vi "LaserPIDPositioning.vi"(0 "Servo Device In":i32, 1 "Vertical Edge":T1 {"Point2 (Real-World)"."Y" format="%.2f"; "Point2 (Real-World)"."X" format="%.2f"; "Point1 (Real-World)"."Y" format="%.2f"; "Point1 (Real-World)"."X" format="%.2f"; "Point2 (Pixels)"."Y" format="%.2f"; "Point2 (Pixels)"."X" format="%.2f"; "Point1 (Pixels)"."Y" format="%.2f"; "Point1 (Pixels)"."X" format="%.2f"}, 2 "Horizontal Edge":T1 {"Point2 (Real-World)"."Y" format="%.2f"; "Point2 (Real-World)"."X" format="%.2f"; "Point1 (Real-World)"."Y" format="%.2f"; "Point1 (Real-World)"."X" format="%.2f"; "Point2 (Pixels)"."Y" format="%.2f"; "Point2 (Pixels)"."X" format="%.2f"; "Point1 (Pixels)"."Y" format="%.2f"; "Point1 (Pixels)"."X" format="%.2f"}, 4 "servo error in":errorcluster, 5 "error in":errorcluster, 8 "Destination Point":cluster{"DestinationX":dbl, "DestinationY":dbl}, 9 "Servo Angles In":cluster{"Angle X":dbl, "Angle Y":dbl}) -> (11 "Servo Angles Out":cluster{"Angle X":dbl, "Angle Y":dbl}, 14 "Servo Device Out":i32, 18 "servo error out":errorcluster, 19 "error out":errorcluster)   [LabVIEW 2014]
uses:
  <vilib>/addons/control/pid/pid.llb/PID (DBL).vi
  <vilib>/vision/NI_Vision_Development_Module.lvlib
  <vilib>/addons/control/pid/NI_PID_pid.lvlib
panel:
  out "x+y 2":dbl
  out "x+y":dbl
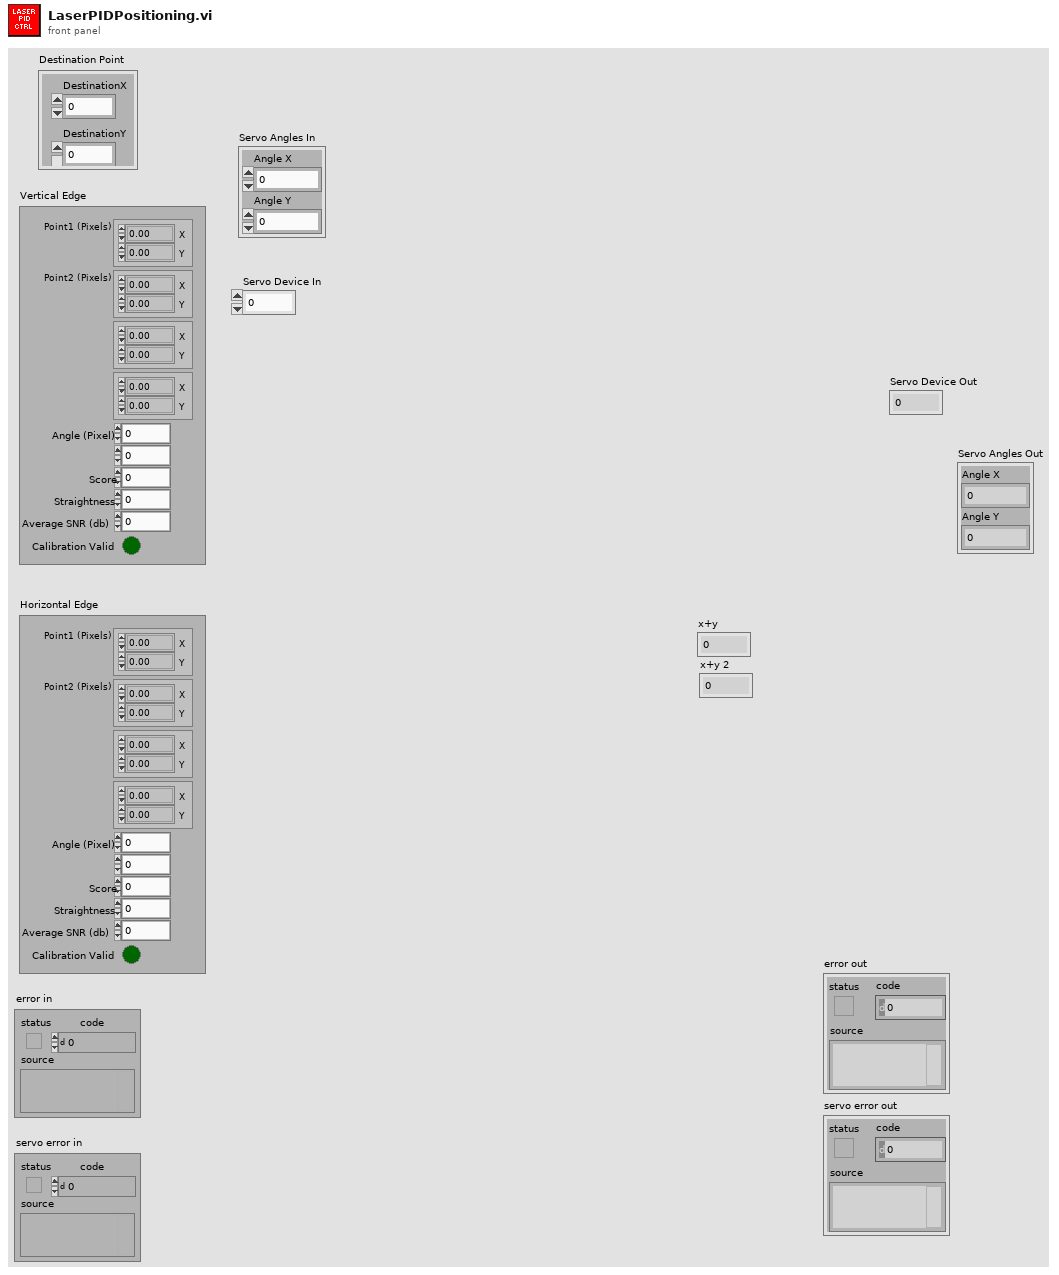
[diagram p1: front panel]
types:
  T1 = cluster{"Point1 (Pixels)":cluster{"X":sgl, "Y":sgl}, "Point2 (Pixels)":cluster{"X":sgl, "Y":sgl}, "Point1 (Real-World)":cluster{"X":sgl, "Y":sgl}, "Point2 (Real-World)":cluster{"X":sgl, "Y":sgl}, "Angle (Pixel)":dbl, "Angle (Real-World)":dbl, "Score":dbl, "Straightness":dbl, "Average SNR (db)":dbl, "Calibration Valid":bool}
  T2 = cluster{"proportional gain (Kc)":dbl, "integral time (Ti, min)":dbl, "derivative time (Td, min)":dbl}
  T3 = cluster{cluster{"X":sgl, "Y":sgl}, cluster{"X":sgl, "Y":sgl}}
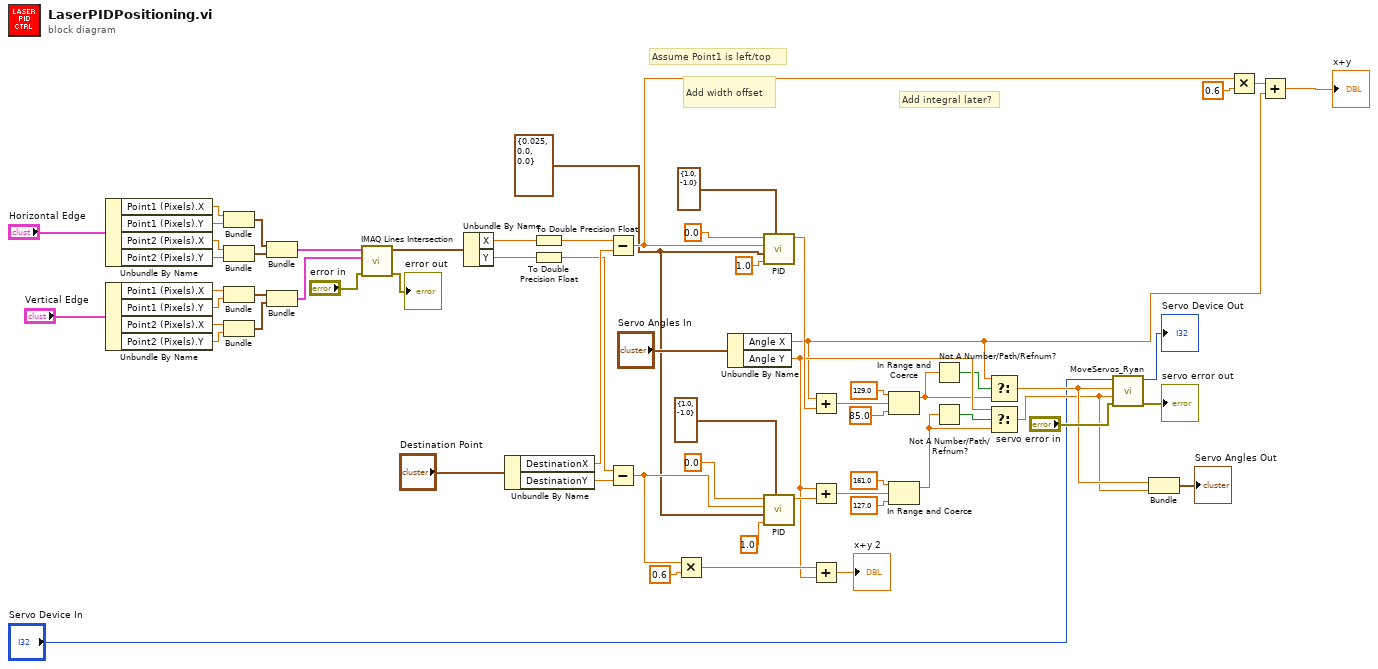
[diagram p0: block diagram]
diagram:
  w1 = T2 {"proportional gain (Kc)"=0.025, "integral time (Ti, min)"=0.0, "derivative time (Td, min)"=0.0} ("PID gains")
  # "Add integral later?"
  # "Add width offset"
  # "Assume Point1 is left/top"
  n1 = Unbundle By Name("Horizontal Edge") -> ("Point1 (Pixels).X"=w60:sgl, "Point1 (Pixels).Y"=w59:sgl, "Point2 (Pixels).X"=w58:sgl, "Point2 (Pixels).Y"=w57:sgl)
  n2 = Unbundle By Name("Vertical Edge") -> ("Point1 (Pixels).X"=w51:sgl, "Point1 (Pixels).Y"=w50:sgl, "Point2 (Pixels).X"=w49:sgl, "Point2 (Pixels).Y"=w48:sgl)
  n3 = Bundle("X"=w60, "Y"=w59) -> (w56:cluster{"X":sgl, "Y":sgl})  [unwired: 1 in]
  n4 = Bundle("X"=w58, "Y"=w57) -> (w55:cluster{"X":sgl, "Y":sgl})  [unwired: 1 in]
  n5 = Bundle("X"=w51, "Y"=w50) -> (w53:cluster{"X":sgl, "Y":sgl})  [unwired: 1 in]
  n6 = Bundle("X"=w49, "Y"=w48) -> (w52:cluster{"X":sgl, "Y":sgl})  [unwired: 1 in]
  n7 = Bundle(w56, w55) -> (w54:T3)  [unwired: 1 in]
  n8 = Bundle(w53, w52) -> (w47:T3)  [unwired: 1 in]
  n9 = call "IMAQ Lines Intersection"("error in (no error)"="error in", "Line 2"=w47, "Line 1"=w54) -> ("error out"=→"error out":errorcluster, "Intersection Point"=w45:cluster{"X":sgl, "Y":sgl})  [unwired: 6 in, 1 out]
  n10 = Unbundle By Name(w45) -> ("X"=w35:sgl, "Y"=w39:sgl)
  n11 = Unbundle By Name("Destination Point") -> ("DestinationX"=w42:dbl, "DestinationY"=w38:dbl)
  n12 = To Double Precision Float(number=w35) -> (double precision float=w24:dbl)
  n13 = To Double Precision Float(number=w39) -> (double precision float=w34:dbl)
  n14 = Subtract(x=w24, y=w42) -> (x-y=w22:dbl)
  n15 = Subtract(x=w34, y=w38) -> (x-y=w19:dbl)
  n16 = Multiply(x=w19, y=0.6) -> (x*y=w18:dbl)
  n17 = Unbundle By Name("Servo Angles In") -> ("Angle X"=w7:dbl, "Angle Y"=w10:dbl)
  n18 = call-poly <vilib>:"PID.vi"("output range"=cluster{"output high":dbl, "output low":dbl} {"output high"=1.0, "output low"=-1.0}, "dt (s)"=1.0, "PID gains"=w1, "process variable"=w22, "setpoint"=0.0) -> ("output"=w13:dbl)  [unwired: 5 in, 1 out]
  n19 = call-poly <vilib>:"PID.vi"("output range"=cluster{"output high":dbl, "output low":dbl} {"output high"=1.0, "output low"=-1.0}, "dt (s)"=1.0, "PID gains"=w1, "process variable"=w19, "setpoint"=0.0) -> ("output"=w15:dbl)  [unwired: 5 in, 1 out]
  n20 = Add(x=w7, y=w13) -> (x+y=w12:dbl)
  n21 = Add(x=w10, y=w15) -> (x+y=w14:dbl)
  n22 = Add(x=w18, y=w10) -> (x+y=→"x+y 2":dbl)
  n23 = In Range and Coerce(upper limit=129.0, x=w12, lower limit=85.0) -> (coerced(x)=w6:dbl)  [unwired: 1 out]
  n24 = In Range and Coerce(upper limit=161.0, x=w14, lower limit=127.0) -> (coerced(x)=w9:dbl)  [unwired: 1 out]
  n25 = Not A Number/Path/Refnum?(number/path/refnum=w6) -> (NaN/Path/Refnum?=w8:bool)
  n26 = Not A Number/Path/Refnum?(number/path/refnum=w9) -> (NaN/Path/Refnum?=w11:bool)
  n27 = Select(t=w7, s=w8, f=w6) -> (s? t:f=w5:dbl)
  n28 = Select(t=w10, s=w11, f=w9) -> (s? t:f=w4:dbl)
  n29 = call "MoveServos_Ryan.vi"("servo error in"="servo error in", "Y pos"=w4, "X pos"=w5, "Device In"="Servo Device In") -> ("servo error out"=→"servo error out":errorcluster, "Device Out"=→"Servo Device Out":i32)  [unwired: 6 in]
  n30 = Bundle("upper limit"=w5, "upper limit"=w4) -> (→"Servo Angles Out":cluster{"upper limit":dbl, "upper limit":dbl})  [unwired: 1 in]
  n31 = Multiply(x=w22, y=0.6) -> (x*y=w21:dbl)
  n32 = Add(x=w21, y=w7) -> (x+y=→"x+y":dbl)
